vi "set_stimulation_only.vi"(8 "error in (no error)":errorcluster, 10 "stimulation only?":bool, 11 "IntrinsicImagingMG091001 in":refnum<class "DataCollectionMG091001IntrinsicImaging.lvclass">) -> (0 "error out":errorcluster, 3 "IntrinsicImagingMG091001 out":refnum<class "DataCollectionMG091001IntrinsicImaging.lvclass">)   [LabVIEW 2010, in "DataCollectionMG091001IntrinsicImaging.lvclass"]
uses:
  DataCollectionMG091001IntrinsicImaging.lvclass
  DataCollectionMG091001IntrinsicImaging.lvclass/DataCollectionMG091001IntrinsicImaging.ctl
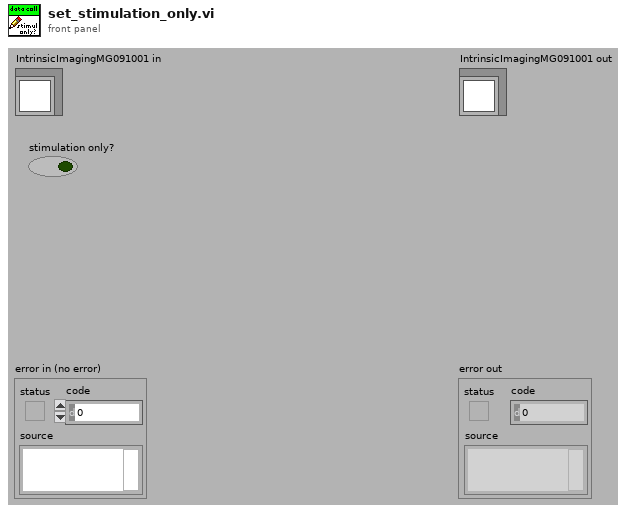
[diagram p1: front panel]
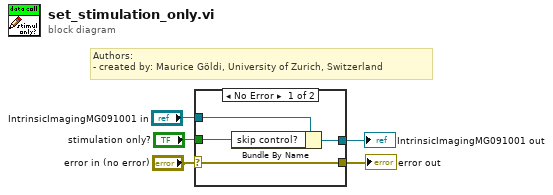
[diagram p0: block diagram]
diagram:
  # "Authors: \n- created by: Maurice Göldi, University of Zurich, Switzerland"
  n1 = case shown="No Error" "error in (no error)" {
    selector: "error in (no error)" -> [w9 w10]
    tunnel: [w9 w10] -> w4
    tunnel: [w7 w11] -> w2
    tunnel: "IntrinsicImagingMG091001 in" -> [w8 w11]
    tunnel: "stimulation only?" -> [w6 _]
    frame No Error {
      n2 = Bundle By Name(cluster=w8, "skip control?"=w6) -> (w7:refnum<class "DataCollectionMG091001IntrinsicImaging.lvclass">)
    }
    frame Error {
    }
  }
  "error out" <- w4
  "IntrinsicImagingMG091001 out" <- w2
